vi "globals.vi"() -> ()   [LabVIEW 2020]
panel:
  out "Delta Theta (deg)":dbl
  out "Robot Position X (in)":dbl
  out "Robot Position Y (in)":dbl
  out "Gyro Theta (deg)":dbl
  out "Gyro Raw (deg)":dbl
  out "EncoderBR":dbl
  out "Encoder BL":dbl
  out "Encoder FL":dbl
  out "Encoder FR":dbl
  out "Drive Target BR":dbl
  out "Azimuth Target BR":dbl
  out "Drive Target BL":dbl
  out "Azimuth Target BL":dbl
  out "Drive Target FL":dbl
  out "Azimuth Target FL":dbl
  out "Azimuth Target FR":dbl
  out "Drive Target FR":dbl
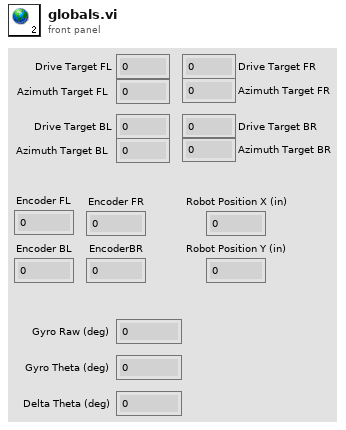
[diagram p1: front panel]
diagram:
